vi "MHM Get Last Error.vi"(8 "error in (no error)":errorcluster, 11 "ulMHMHandle":u32) -> (0 "error out":errorcluster, 1 "pulErrorType":u32, 2 "pulLastError":u32, 3 "function return":u32, 5 "pcErrorText":string)   [LabVIEW 2017, in "MHM_1SL_interface.lvlib"]
uses:
  MHM_1SL_interface.lvlib
  SSI_Tool/DUT_Interface/lv_interface/lib/MHM_1SL_interface.dll
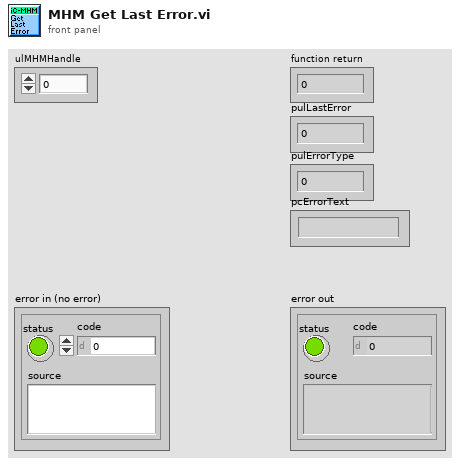
[diagram p1: front panel]
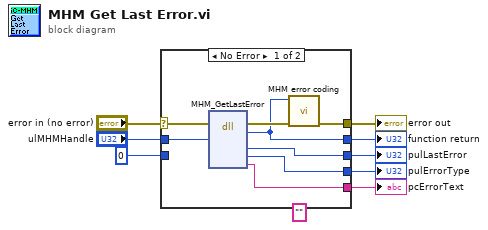
[diagram p0: block diagram]
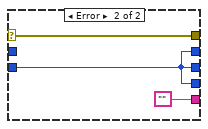
[diagram p2: hidden frame]
diagram:
  n1 = case shown="No Error" "error in (no error)" {
    selector: "error in (no error)" -> [w16 w19]
    tunnel: "ulMHMHandle" -> [w15 _]
    tunnel: [w13 w19] -> w6
    tunnel: [w12 w18] -> w5
    tunnel: [w11 w18] -> w4
    tunnel: [w10 w18] -> w3
    tunnel: [w9 ""] -> w2
    tunnel: u32 0 -> [_ w18]
    frame No Error {
      (unwired) "" ("pcErrorText")
      n2 = dll-call lib="C:/workspace/project/scancon/sw/SSI_Tool/DUT_Interface/lv_interface/lib/MHM_1SL_interface.dll" fn="MHM_GetLastError"(error in=w16, "ulMHMHandle"=w15) -> (error out=w14:errorcluster, "return type"=w12:u32, "pulLastError"=w11:u32, "pulErrorType"=w10:u32, "pcErrorText"=w9:string)  [unwired: 6 in, 1 out]
      n3 = call "MHM error coding.vi"("error in (no error)"=w14, "function return in"=w12) -> ("error out"=w13:errorcluster)  [unwired: 9 in]
    }
    frame Error {
    }
  }
  "function return" <- w5
  "error out" <- w6
  "pulLastError" <- w4
  "pulErrorType" <- w3
  "pcErrorText" <- w2
